vi "Cleanup.vi"(8 "error in (no error)":errorcluster, 10 "Owner":refnum<vi>, 11 "vi refnum":refnum<vi>) -> (0 "error out":errorcluster, 3 "Type out":variant)   [LabVIEW 2018, in "JSON to LVConstant Test.lvlib"]
uses:
  JSON to LVConstant Test.lvlib
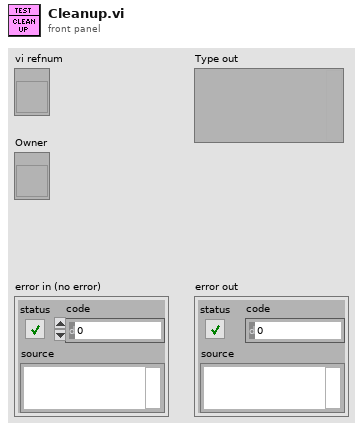
[diagram p1: front panel]
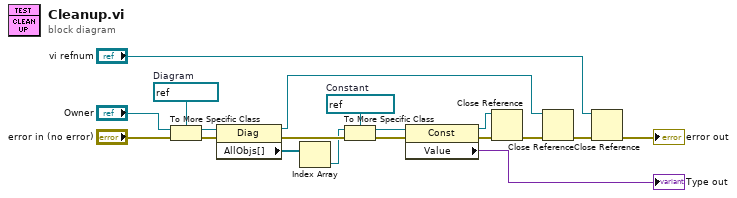
[diagram p0: block diagram]
diagram:
  w16 = refnum<vi> refnum  # Constant
  w10 = refnum<vi> refnum  # Diagram
  n1 = To More Specific Class(target class=w10, reference="Owner", error in="error in (no error)") -> (specific class reference=w9:refnum<vi>, error out=w7:errorcluster)
  n2 = property on="Property Node" class="Diag"(reference=w9, error in=w7) -> (reference out=w6:refnum<vi>, error out=w19:errorcluster, "AllObjs[]"=w11:refnum<vi>[])
  n3 = Index Array(array=w11) -> (element=w14:refnum<vi>)  [unwired: 1 in]
  n4 = To More Specific Class(target class=w16, reference=w14, error in=w19) -> (specific class reference=w15:refnum<vi>, error out=w13:errorcluster)
  n5 = property on="Property Node" class="Const"(reference=w15, error in=w13) -> (reference out=w17:refnum<vi>, error out=w12:errorcluster, "Value"=→"Type out":variant)
  n6 = Close Reference(reference=w17, error in (no error)=w12) -> (error out=w18:errorcluster)
  n7 = Close Reference(reference=w6, error in (no error)=w18) -> (error out=w4:errorcluster)
  n8 = Close Reference(reference="vi refnum", error in (no error)=w4) -> (error out=→"error out":errorcluster)
